vi "Replace Icon Layer.vi"() -> ()   [LabVIEW 2015]
doc: "<b> </b> <b> </b>\n©2016 Q Software Innovations, LLC (QSI)\nwritten by Quentin Alldredge\nproduced in LabVIEW 2015"
uses:
  <vilib>/LabVIEW Icon API/lv_icon/Classes/Layer/Layer.lvclass
  <vilib>/LabVIEW Icon API/lv_icon/Controls/Layer.ctl
  <vilib>/LabVIEW Icon API/lv_icon/Classes/Icon/Icon.lvclass
  Project Manipulation Scripts/Project Manipulation Scripts.lvlib
  <vilib>/LabVIEW Icon API/LabVIEW Icon API.lvlib
panel:
  out "LayerIcon":picture
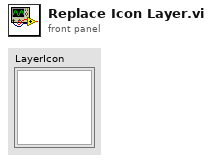
[diagram p1: front panel]
types:
  T1 = typedef "Layer.ctl" = cluster{"LayerIcon":picture, "LayerName":string, "Opacity":u8, "Visibility?":bool}
  T2 = typedef "imagedata.ctl" = cluster{"image type":i32, "image depth":i32, "image":u8[], "mask":u8[], "colors":u32[], "Rectangle":cluster{"left":i16, "top":i16, "right":i16, "bottom":i16}}
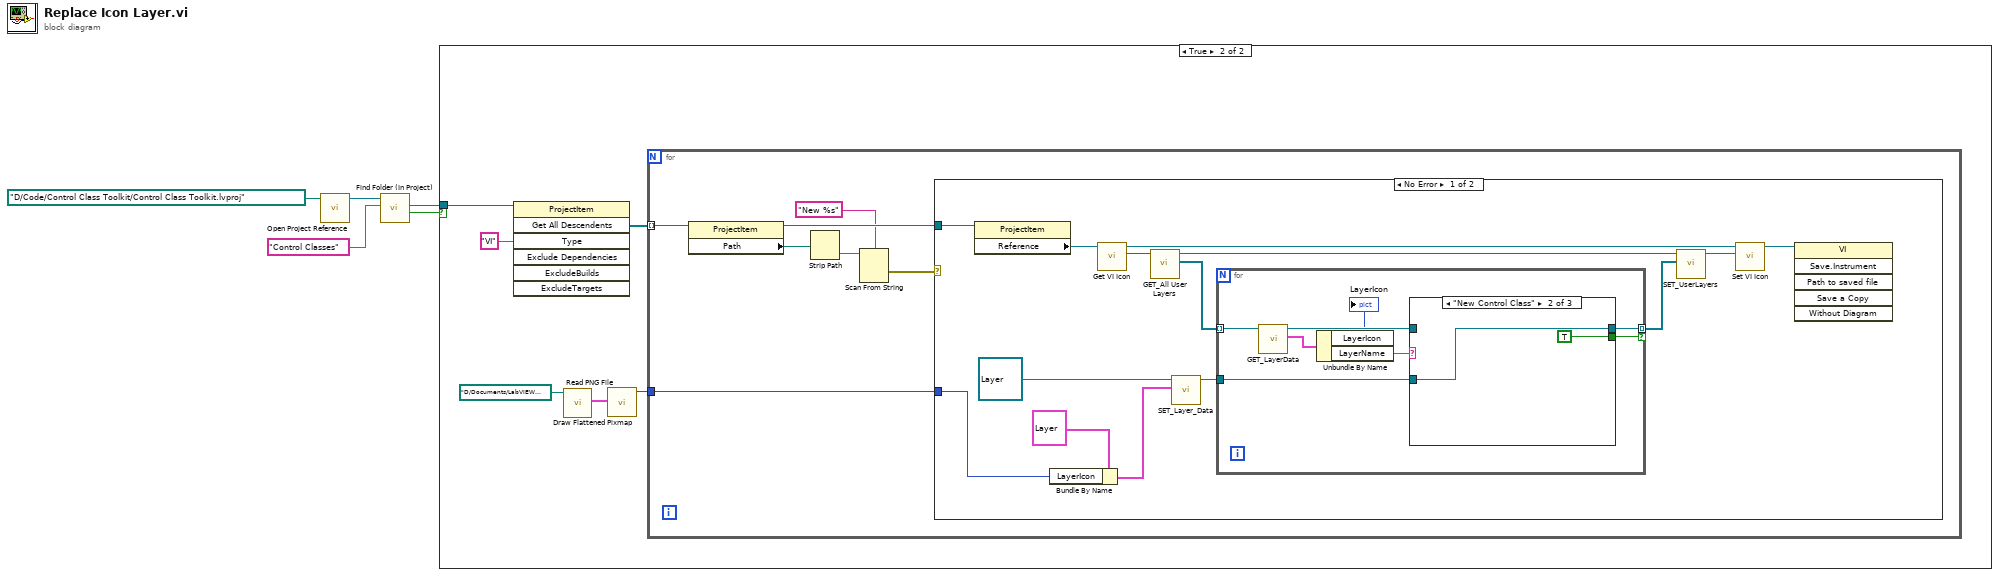
[diagram p0: block diagram]
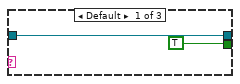
[diagram p3: hidden frame]
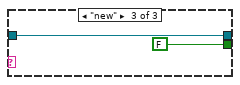
[diagram p4: hidden frame]
diagram:
  n1 = call "Open Project Reference.vi"("Project Path"=path "D:/Code/Control Class Toolkit/Control Class Toolkit.lvproj") -> ("Project out"=w4:refnum<vi>)  [unwired: 10 in]
  n2 = call "Find Folder (In Project).vi"("Folder Name"="Control Classes", "Project in"=w4) -> ("Found?"=w2:bool, "Folder Refnum"=w1:refnum<vi>)  [unwired: 7 in, 1 out]
  n3 = case shown="True" w2 {
    tunnel: w1 -> [_ w11]
    frame False {
    }
    frame True {
      n4 = invoke class="ProjectItem" method="Get All Descendents"(reference=w11, "Type"="VI") -> ("All Descendents"=w9:refnum<vi>[])  [unwired: 5 in, 6 out]
      n5 = call <vilib>:"Read PNG File.vi"("path to PNG file"=path "D:/Documents/LabVIEW Data/Glyphs/New Control Class.png") -> ("image data"=w7:T2)  [unwired: 8 in, 2 out]
      n6 = call <vilib>:"Draw Flattened Pixmap.vi"("image data"=w7) -> ("new picture"=w6:picture)  [unwired: 8 in]
      n7 = for {
        tunnel: w9 -> [w18] mode=indexing
        tunnel: w6 -> [w15]
        n8 = property class="ProjectItem"(reference=w18) -> (reference out=w16:refnum<vi>, "Path"=w17:path)  [unwired: 1 in, 1 out]
        n9 = Strip Path(path=w17) -> (name=w14:string)  [unwired: 1 out]
        n10 = Scan From String(format string="New %s", input string=w14) -> (error out=w13:errorcluster)  [unwired: 4 in, 2 out]
        n11 = case shown="No Error" w13 {
          tunnel: w16 -> [w32 _]
          tunnel: w15 -> [w19 _]
          frame No Error {
            n12 = property class="ProjectItem"(reference=w32) -> ("Reference"=w31:refnum<vi>)  [unwired: 1 in, 2 out]
            n13 = Bundle By Name(cluster=T1 {"LayerIcon"=bytes[3102], "LayerName"="New Control Class", "Opacity"=100, "Visibility?"=TRUE} ("Data"), "LayerIcon"=w19) -> (w26:T1)
            n14 = call <vilib>:"Get VI Icon.vi"("VI Refnum in"=w31) -> ("Icon"=w30:refnum<class "Icon.lvclass">, "VI Refnum out"=w21:refnum<vi>)  [unwired: 8 in, 1 out]
            n15 = call-dynamic "GET_All User Layers.vi"("Icon.lvclass in"=w30) -> ("User Layer"=w29:refnum<class "Layer.lvclass">[], "Icon.lvclass out"=w23:refnum<class "Icon.lvclass">)  [unwired: 8 in, 1 out]
            n16 = call-dynamic "SET_Layer_Data.vi"("Data"=w26, "Layer.lvclass in"=refnum<class "Layer.lvclass"> refnum ("Layer.lvclass")) -> ("Layer.lvclass out"=w25:refnum<class "Layer.lvclass">)  [unwired: 8 in, 1 out]
            n17 = for {
              tunnel: w29 -> [w40] mode=indexing
              tunnel: [w36] -> w24 mode=indexing if=w33
              tunnel: w25 -> [w35]
              n18 = call-dynamic "GET_LayerData.vi"("Layer.lvclass in"=w40) -> ("Data"=w39:T1, "Layer.lvclass out"=w38:refnum<class "Layer.lvclass">)  [unwired: 6 in, 3 out]
              n19 = Unbundle By Name(w39) -> ("LayerIcon"=→"LayerIcon":picture, "LayerName"=w37:string)
              n20 = case shown="\"New Control Class\"" w37 {
                tunnel: w38 -> [w42 _ w46]
                tunnel: [w42 w44 w46] -> w36
                tunnel: w35 -> [_ w44 _]
                tunnel: [TRUE TRUE FALSE] -> w33
                frame Default {
                }
                frame "New Control Class" {
                }
                frame "new" {
                }
              }
            }
            n21 = call-dynamic "SET_UserLayers.vi"("Layers"=w24, "Icon.lvclass in"=w23) -> ("Icon.lvclass out"=w22:refnum<class "Icon.lvclass">)  [unwired: 8 in, 1 out]
            n22 = call <vilib>:"Set VI Icon.vi"("Icon"=w22, "VI Refnum in"=w21) -> ("VI Refnum out"=w20:refnum<vi>)  [unwired: 8 in, 1 out]
            n23 = invoke class="VI" method="Save.Instrument"(reference=w20) -> ()  [unwired: 5 in, 6 out]
          }
          frame Error {
          }
        }
      }
    }
  }
